vi "Read X.vi"(8 "error in (no error)":errorcluster, 11 "MarkAbs in":refnum<class "MarkAbs.lvclass">) -> (0 "error out":errorcluster, 2 "X":dbl, 3 "MarkAbs out":refnum<class "MarkAbs.lvclass">)   [LabVIEW 2013, in "HardwareCharacterization.lvlib" / "MarkAbs.lvclass"]
uses:
  MarkAbs.lvclass
  MarkAbs.lvclass/MarkAbs.ctl
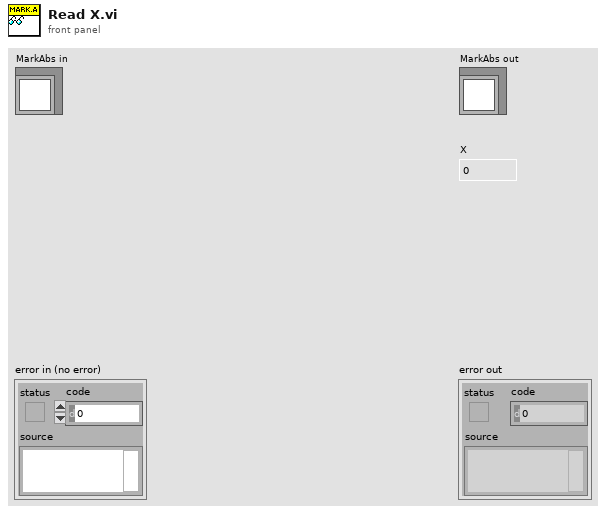
[diagram p1: front panel]
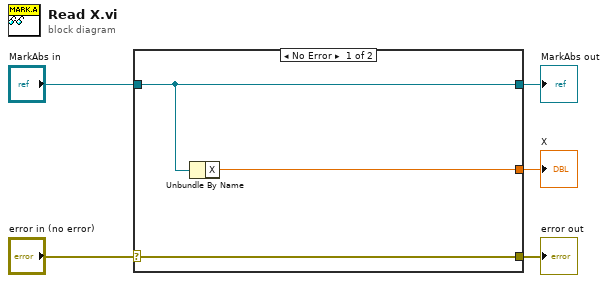
[diagram p0: block diagram]
diagram:
  n1 = case shown="No Error" "error in (no error)" {
    selector: "error in (no error)" -> [w8 w9]
    tunnel: [w8 w9] -> w4
    tunnel: [w7 w10] -> w2
    tunnel: "MarkAbs in" -> [w7 w10]
    tunnel: [w6 _] -> w1
    frame No Error {
      n2 = Unbundle By Name(w7) -> ("X"=w6:dbl)
    }
    frame Error {
    }
  }
  "error out" <- w4
  "MarkAbs out" <- w2
  "X" <- w1
